vi "AddUser2.vi"(3 "Add?":bool) -> (0 "password":string, 1 "login":string, 2 "Success?":bool)   [LabVIEW 2016]
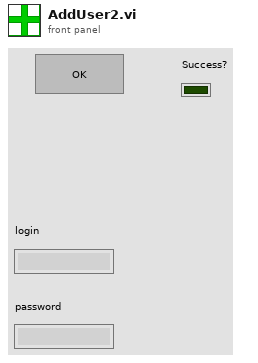
[diagram p1: front panel]
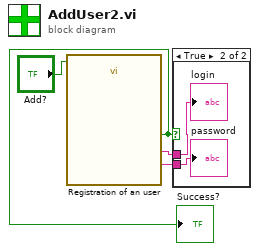
[diagram p0: block diagram]
diagram:
  n1 = call "Registration of an user"("Enable"="Add?") -> ("Password"=w2:string, "Login"=w3:string, "Input"=w1:bool)  [unwired: 15 in, 1 out]
  "Success?" <- w1
  n2 = case shown="True" w1 {
    tunnel: w3 -> [_ w5]
    tunnel: w2 -> [_ w6]
    frame False {
    }
    frame True {
      "login" <- w5
      "password" <- w6
    }
  }
